vi "WPI_RobotDriveOpen4Motor.vi"   [LabVIEW 2025]
doc: "Opens a reference to the robot drive for a four-motor robot using a choice from supported motor controllers or \"Exisiting\" motor controllers. Robot Drive Open configures all four motors (with the exception of <B>Existing Motors</B>). You must open a reference before using any other VIs on this palette.\n\nThis software is licensed. Open the labview\\readme\\WPI Robotics Library Open Source License.txt file for more information."
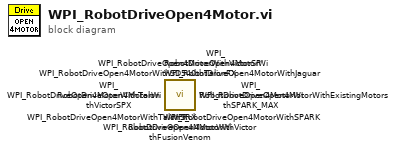
[diagram p0: block diagram]
diagram:
  n1 = call <vilib>:"WPI_RobotDriveOpen4MotorWithFusionVenom.vi"() -> ()  [unwired: 14 in, 2 out]
  n2 = call <vilib>:"WPI_RobotDriveOpen4MotorWithTalonFX.vi"() -> ()  [unwired: 14 in, 2 out]
  n3 = call <vilib>:"WPI_RobotDriveOpen4MotorWithVictorSPX.vi"() -> ()  [unwired: 14 in, 2 out]
  n4 = call <vilib>:"WPI_RobotDriveOpen4MotorWithSPARK_MAX.vi"() -> ()  [unwired: 14 in, 2 out]
  n5 = call <vilib>:"WPI_RobotDriveOpen4MotorWithSD540.vi"() -> ()  [unwired: 14 in, 2 out]
  n6 = call <vilib>:"WPI_RobotDriveOpen4MotorWithSPARK.vi"() -> ()  [unwired: 14 in, 2 out]
  n7 = call <vilib>:"WPI_RobotDriveOpen4MotorWithTalonSRX.vi"() -> ()  [unwired: 14 in, 2 out]
  n8 = call <vilib>:"WPI_RobotDriveOpen4MotorWithVictorSP.vi"() -> ()  [unwired: 14 in, 2 out]
  n9 = call <vilib>:"WPI_RobotDriveOpen4MotorWithTalon.vi"() -> ()  [unwired: 14 in, 2 out]
  n10 = call <vilib>:"WPI_RobotDriveOpen4MotorWithExistingMotors.vi"() -> ()  [unwired: 14 in, 2 out]
  n11 = call <vilib>:"WPI_RobotDriveOpen4MotorWithVictor.vi"() -> ()  [unwired: 14 in, 2 out]
  n12 = call <vilib>:"WPI_RobotDriveOpen4MotorWithJaguar.vi"() -> ()  [unwired: 14 in, 2 out]
